vi "QFGV.vi"(8 "error in (no error)":errorcluster, 11 "QName":string) -> (0 "error out":errorcluster, 3 "ModuleQ":refnum<queue>)   [LabVIEW 2020, in "Template.lvlib"]
doc: "FGV holding reference to the Q of the owning module"
uses:
  Template.lvlib
  Controls/QMessage.ctl
  Controls/QGFVMode.ctl
panel:
  in  "Mode":T1=enum."Get"
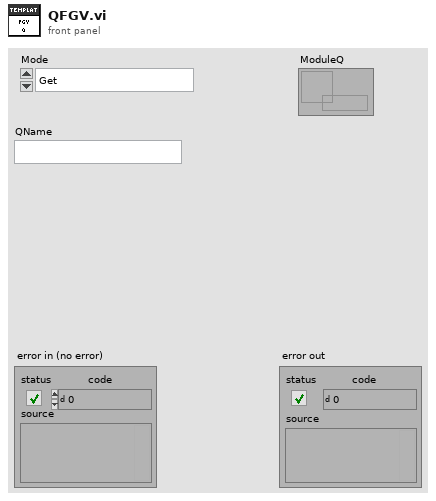
[diagram p1: front panel]
types:
  T1 = typedef "Template.lvlib/QGFVMode.ctl" = enum16{"Create", "Get", "Release"}
  T2 = typedef "Template.lvlib/QMessage.ctl" = cluster{"Command":string, "Data":variant}
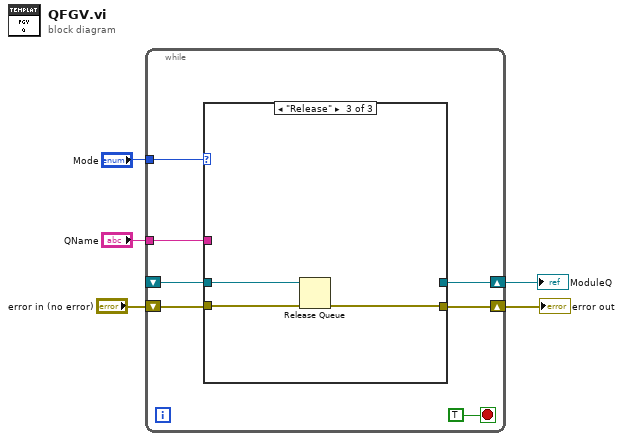
[diagram p0: block diagram]
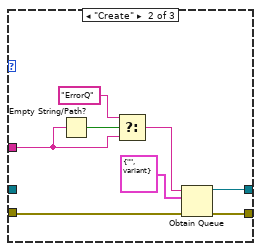
[diagram p3: hidden frame]
diagram:
  n1 = while {
    tunnel: "QName" -> [w10]
    tunnel: "Mode" -> [w8]
    shift-right: [w11] -> w4
    shift-left: "error in (no error)" -> [w12]
    shift-right: [w9] -> w2
    shift-left: _ -> [w6]
    stop <- TRUE stop-if-true
    n2 = case shown="\"Release\"" w8 {
      tunnel: w12 -> [w13 w22 w25]
      tunnel: [w13 w21 w24] -> w11
      tunnel: w10 -> [_ w18 _]
      tunnel: [w14 w15 _] -> w9
      tunnel: w6 -> [w14 _ w23]
      frame Default {
      }
      frame "Create" {
        n3 = Empty String/Path?(string/path=w18) -> (empty?=w20:bool)
        n4 = Select(t="ErrorQ" ("name (unnamed)"), s=w20, f=w18) -> (s? t:f=w17:string)
        n5 = Obtain Queue(name (unnamed)=w17, element data type=T2 {"Command"="", "Data"=variant(errorcluster {"status"=FALSE, "code"=0, "source"=""})}, error in (no error)=w22) -> (queue out=w15:refnum<queue>, error out=w21:errorcluster)  [unwired: 2 in, 1 out]
      }
      frame "Release" {
        n6 = Release Queue(queue=w23, error in (no error)=w25) -> (error out=w24:errorcluster)  [unwired: 1 in, 2 out]
      }
    }
  }
  "error out" <- w4
  "ModuleQ" <- w2
